vi "Stream_data.vi"(0 "VISA resource name in":refnum<visa-resource-name>, 5 "ReadStatus in":refnum<notifier>, 7 "Play / Pause":bool, 9 "Read TTL status in":bool, 11 "error in (no error)":errorcluster, 12 "Notifier error in":errorcluster) -> (4 "VISA Refnum out":refnum<visa-resource-name>, 6 "ReadStatus out":refnum<notifier>, 8 "Read TTL status out":bool, 10 "Current time":timestamp, 13 "VISA error out":errorcluster, 14 "Notifier error out":errorcluster, 15 "read buffer":string)   [LabVIEW 2016]
uses:
  <vilib>/Instr/_visa.llb/VISA Flush IO Buffer Mask.ctl
  Globaltracker.vi
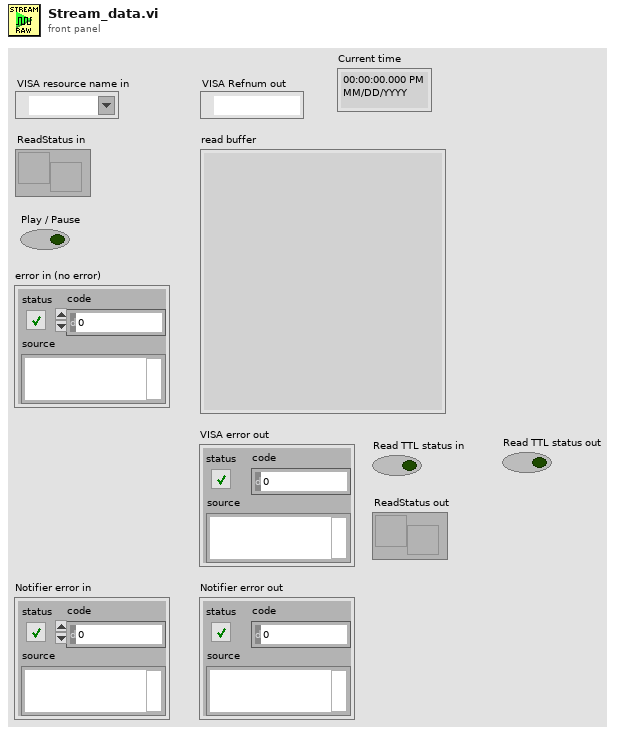
[diagram p1: front panel]
types:
  T1 = typedef "VISA Flush IO Buffer Mask.ctl" = u16
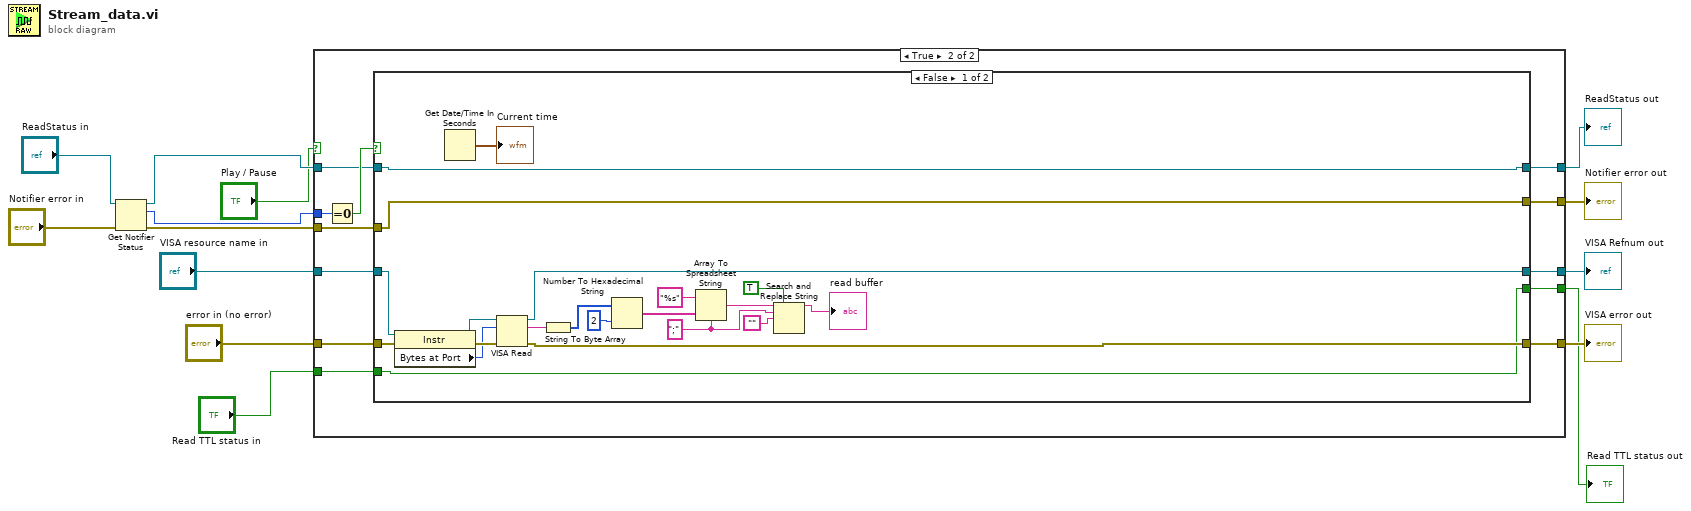
[diagram p0: block diagram]
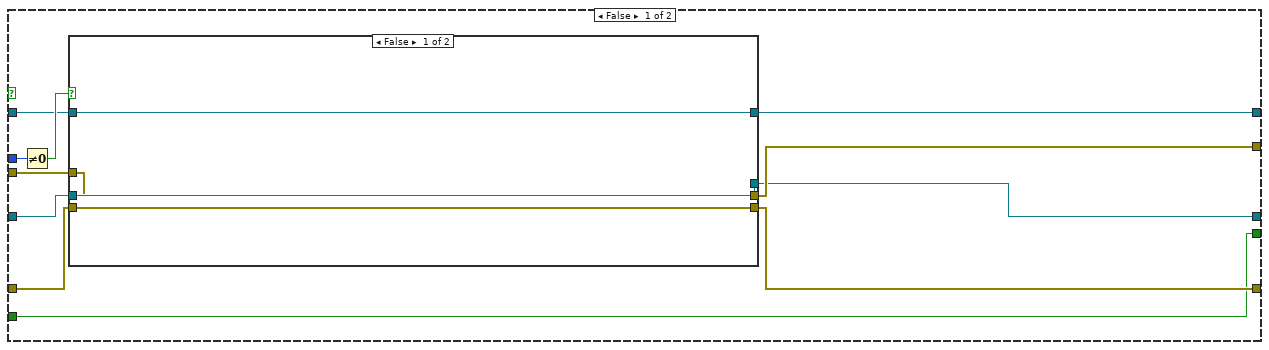
[diagram p2: hidden frame]
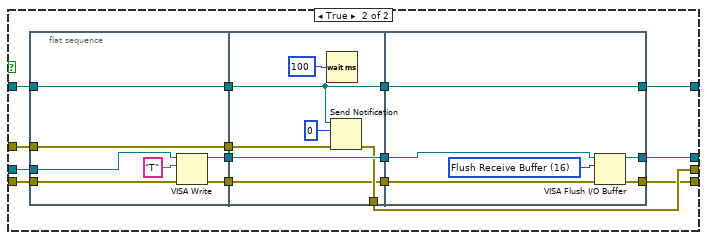
[diagram p3: hidden frame]
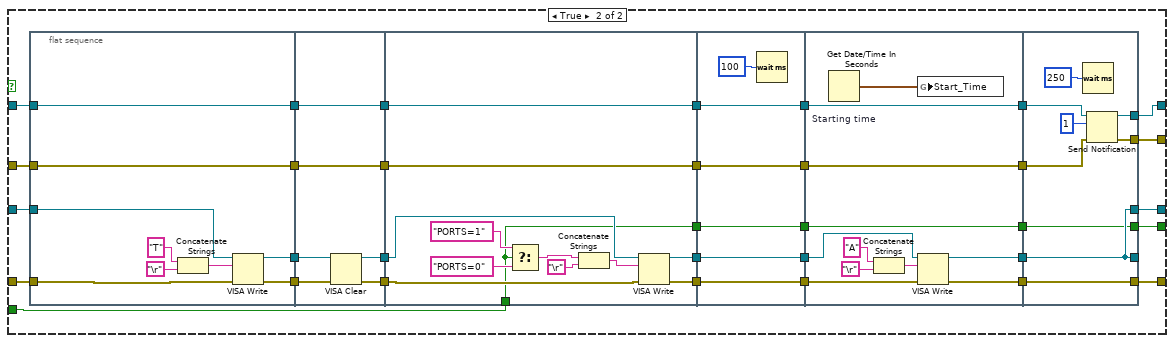
[diagram p4: hidden frame]
diagram:
  n1 = Get Notifier Status(notifier="ReadStatus in", error in (no error)="Notifier error in") -> (notifier out=w11:refnum<notifier>, current notification=w14:i32, error out=w12:errorcluster)  [unwired: 2 out]
  n2 = case shown="True" "Play / Pause" {
    tunnel: [w17 w68] -> w4
    tunnel: [w18 w69] -> w5
    tunnel: w14 -> [w25 w75]
    tunnel: "error in (no error)" -> [w23 w74]
    tunnel: "VISA resource name in" -> [w22 w73]
    tunnel: w11 -> [w21 w72]
    tunnel: w12 -> [w20 w71]
    tunnel: [w19 w70] -> w13
    tunnel: "Read TTL status in" -> [w15 w67]
    tunnel: [w16 w66] -> w2
    tunnel: [w15 w65] -> w1
    frame False {
      n3 = Not Equal To 0?(x=w25) -> (x != 0?=w24:bool)
      n4 = case shown="False" w24 {
        tunnel: w23 -> [w29 w40]
        tunnel: w22 -> [w28 w39]
        tunnel: w21 -> [w26 w38]
        tunnel: w20 -> [w27 w37]
        tunnel: [w27 w36] -> w19
        tunnel: [w28 w35] -> w18
        tunnel: [w29 w34] -> w17
        tunnel: [w26 w31] -> w16
        frame False {
        }
        frame True {
          n5 = flat-sequence {
            tunnel: w39 -> [w51]
            tunnel: w40 -> [w50]
            tunnel: [w49] -> w44
            tunnel: [w48] -> w43
            tunnel: [w47] -> w42
            tunnel: w38 -> [w47]
            tunnel: [w46] -> w41
            tunnel: w37 -> [w46]
            tunnel: w44 -> [w57]
            tunnel: w43 -> [w53]
            tunnel: [w56] -> w36
            tunnel: w42 -> [w52]
            tunnel: w41 -> [w55]
            tunnel: [w57] -> w33
            tunnel: [w53] -> w32
            tunnel: [w52] -> w30
            tunnel: [w64] -> w34
            tunnel: [w61] -> w35
            tunnel: w33 -> [w62]
            tunnel: w32 -> [w63]
            tunnel: [w59] -> w31
            tunnel: w30 -> [w59]
            frame #0 {
              n6 = VISA Write(VISA resource name=w51, write buffer="T", error in (no error)=w50) -> (VISA resource name out=w49:refnum<visa-resource-name>, error out=w48:errorcluster)  [unwired: 1 out]
            }
            frame #1 {
              n7 = Wait (ms)(milliseconds to wait=u32 100) -> ()  [unwired: 1 out]
              n8 = Send Notification(notification=0, notifier=w52, error in (no error)=w55) -> (error out=w56:errorcluster)  [unwired: 1 out]
            }
            frame #2 {
              w60 = T1 16 items=["Flush Receive Buffer"=16, "Write Transmit Buffer to Device"=32, "Flush Receive Buffer (No I/O)"=64, "Flush Transmit Buffer"=128] ("Mask")
              n9 = VISA Flush I/O Buffer(VISA resource name=w62, mask (16)=w60, error in (no error)=w63) -> (VISA resource name out=w61:refnum<visa-resource-name>, error out=w64:errorcluster)
            }
          }
        }
      }
    }
    frame True {
      n10 = Equal To 0?(x=w75) -> (x = 0?=w76:bool)
      n11 = case shown="False" w76 {
        tunnel: w74 -> [w97 w126]
        tunnel: w73 -> [w96 w125]
        tunnel: w72 -> [w78 w124]
        tunnel: w71 -> [w90 w123]
        tunnel: [w90 w122] -> w70
        tunnel: [w92 w121] -> w69
        tunnel: [w91 w120] -> w68
        tunnel: w67 -> [w77 w111]
        tunnel: [w78 w110] -> w66
        tunnel: [w77 w101] -> w65
        frame False {
          w84 = ";" ("delimiter (Tab)")
          n12 = property class="Instr"(reference=w96, error in=w97) -> (reference out=w95:refnum<visa-resource-name>, error out=w94:errorcluster, "Bytes at Port"=w93:u32)
          n13 = Get Date/Time In Seconds ("Current time")() -> (seconds since 1Jan1904=→"Current time":timestamp)
          n14 = VISA Read(VISA resource name=w95, byte count=w93, error in (no error)=w94) -> (VISA resource name out=w92:refnum<visa-resource-name>, read buffer=w82:string, error out=w91:errorcluster)  [unwired: 1 out]
          n15 = String To Byte Array(string=w82) -> (unsigned byte array=w89:u8[])
          n16 = Number To Hexadecimal String(1:i16 2 ("width (-)"), 2:w89) -> (0:w87:string[])
          n17 = Array To Spreadsheet String(delimiter (Tab)=w84, array=w87, 3:"%s" ("format string")) -> (spreadsheet string=w85:string)
          n18 = Search and Replace String(replace all?=TRUE ("replace all? (F)"), input string=w85, search string=w84, replace string="") -> (result string=→"read buffer":string)  [unwired: 4 in, 3 out]
        }
        frame True {
          n19 = flat-sequence {
            tunnel: w126 -> [w135]
            tunnel: w125 -> [w136]
            tunnel: w123 -> [w138]
            tunnel: w124 -> [w139]
            tunnel: [w139] -> w119
            tunnel: [w138] -> w118
            tunnel: [w137] -> w117
            tunnel: [w134] -> w116
            tunnel: [w145] -> w105
            tunnel: [w144] -> w104
            tunnel: [w143] -> w103
            tunnel: [w142] -> w102
            tunnel: w116 -> [w141]
            tunnel: w117 -> [w140]
            tunnel: w118 -> [w144]
            tunnel: w119 -> [w145]
            tunnel: w105 -> [w157]
            tunnel: [w157] -> w115
            tunnel: w104 -> [w156]
            tunnel: [w156] -> w114
            tunnel: w103 -> [w153]
            tunnel: [w152] -> w113
            tunnel: w102 -> [w151]
            tunnel: [w150] -> w112
            tunnel: w111 -> [w146]
            tunnel: [w146] -> w98
            tunnel: [w163] -> w109
            tunnel: [w162] -> w108
            tunnel: [w161] -> w107
            tunnel: [w160] -> w106
            tunnel: w112 -> [w160]
            tunnel: w113 -> [w161]
            tunnel: w114 -> [w162]
            tunnel: w115 -> [w163]
            tunnel: [w158] -> w99
            tunnel: w98 -> [w158]
            tunnel: [w171] -> w130
            tunnel: [w170] -> w129
            tunnel: [w167] -> w128
            tunnel: [w166] -> w127
            tunnel: w109 -> [w171]
            tunnel: w108 -> [w170]
            tunnel: w107 -> [w169]
            tunnel: w106 -> [w168]
            tunnel: [w164] -> w100
            tunnel: w99 -> [w164]
            tunnel: w130 -> [w182]
            tunnel: w129 -> [w181]
            tunnel: [w179] -> w122
            tunnel: [w178] -> w120
            tunnel: w128 -> [w178]
            tunnel: [w177] -> _
            tunnel: w127 -> [w177]
            tunnel: [w177] -> w121
            tunnel: [w176] -> w110
            tunnel: [w175] -> w101
            tunnel: w100 -> [w175]
            frame #0 {
              n20 = Concatenate Strings("T" ("write buffer"), "\r") -> (w131:string)
              n21 = VISA Write(VISA resource name=w136, write buffer=w131, error in (no error)=w135) -> (VISA resource name out=w137:refnum<visa-resource-name>, error out=w134:errorcluster)  [unwired: 1 out]
            }
            frame #1 {
              n22 = VISA Clear(VISA resource name=w140, error in (no error)=w141) -> (VISA resource name out=w143:refnum<visa-resource-name>, error out=w142:errorcluster)
            }
            frame #2 {
              n23 = Select(t="PORTS=1" ("write buffer"), s=w146, f="PORTS=0" ("write buffer")) -> (s? t:f=w149:string)
              n24 = Concatenate Strings(w149, "\r") -> (w154:string)
              n25 = VISA Write(VISA resource name=w153, write buffer=w154, error in (no error)=w151) -> (VISA resource name out=w152:refnum<visa-resource-name>, error out=w150:errorcluster)  [unwired: 1 out]
            }
            frame #3 {
              n26 = Wait (ms)(milliseconds to wait=u32 100) -> ()  [unwired: 1 out]
            }
            frame #4 {
              n27 = Get Date/Time In Seconds "Starting time"() -> (seconds since 1Jan1904=w165:timestamp)
              n28 = Concatenate Strings("A" ("write buffer"), "\r") -> (w172:string)
              n29 = global write "Globaltracker.vi" "Start_Time"(w165) -> ()
              n30 = VISA Write(VISA resource name=w169, write buffer=w172, error in (no error)=w168) -> (VISA resource name out=w166:refnum<visa-resource-name>, error out=w167:errorcluster)  [unwired: 1 out]
            }
            frame #5 {
              n31 = Wait (ms)(milliseconds to wait=u32 250) -> ()  [unwired: 1 out]
              n32 = Send Notification(notification=1, notifier=w182, error in (no error)=w181) -> (notifier out=w176:refnum<notifier>, error out=w179:errorcluster)
            }
          }
        }
      }
    }
  }
  "Notifier error out" <- w13
  "VISA Refnum out" <- w5
  "VISA error out" <- w4
  "ReadStatus out" <- w2
  "Read TTL status out" <- w1
